vi "SI101_ACT_loop_n.vi"(0 "SI101_AverageReactorCoolantTemperature.lvclass in":refnum<class "SI101_AverageReactorCoolantTemperature.lvclass">, 1 "3 JEC10 CT001A XQ01":dbl, 2 "3 JEC20 CT001A XQ01":dbl, 3 "3 JEC30 CT001A XQ01":dbl, 4 "3 JEC40 CT001A XQ01":dbl, 5 "error in (no error)":errorcluster) -> (14 "SI101_AverageReactorCoolantTemperature.lvclass out":refnum<class "SI101_AverageReactorCoolantTemperature.lvclass">, 15 "JEC10CT001A":dbl, 16 "JEC20CT001A":dbl, 17 "JEC30CT001A":dbl, 18 "JEC40CT001A":dbl, 19 "error out":errorcluster)   [LabVIEW 2022 SP3, in "SI101_AverageReactorCoolantTemperature.lvclass"]
uses:
  SI101/SI101_AverageReactorCoolantTemperature.lvclass
  SI101/SI101_AverageReactorCoolantTemperature.lvclass/SI101_AverageReactorCoolantTemperature.ctl
panel:
  in  "Set Params":T1
  in  "Set Params 4":T1
  in  "Set Params 3":T1
  in  "Set Params 2":T1
  # "SI101"
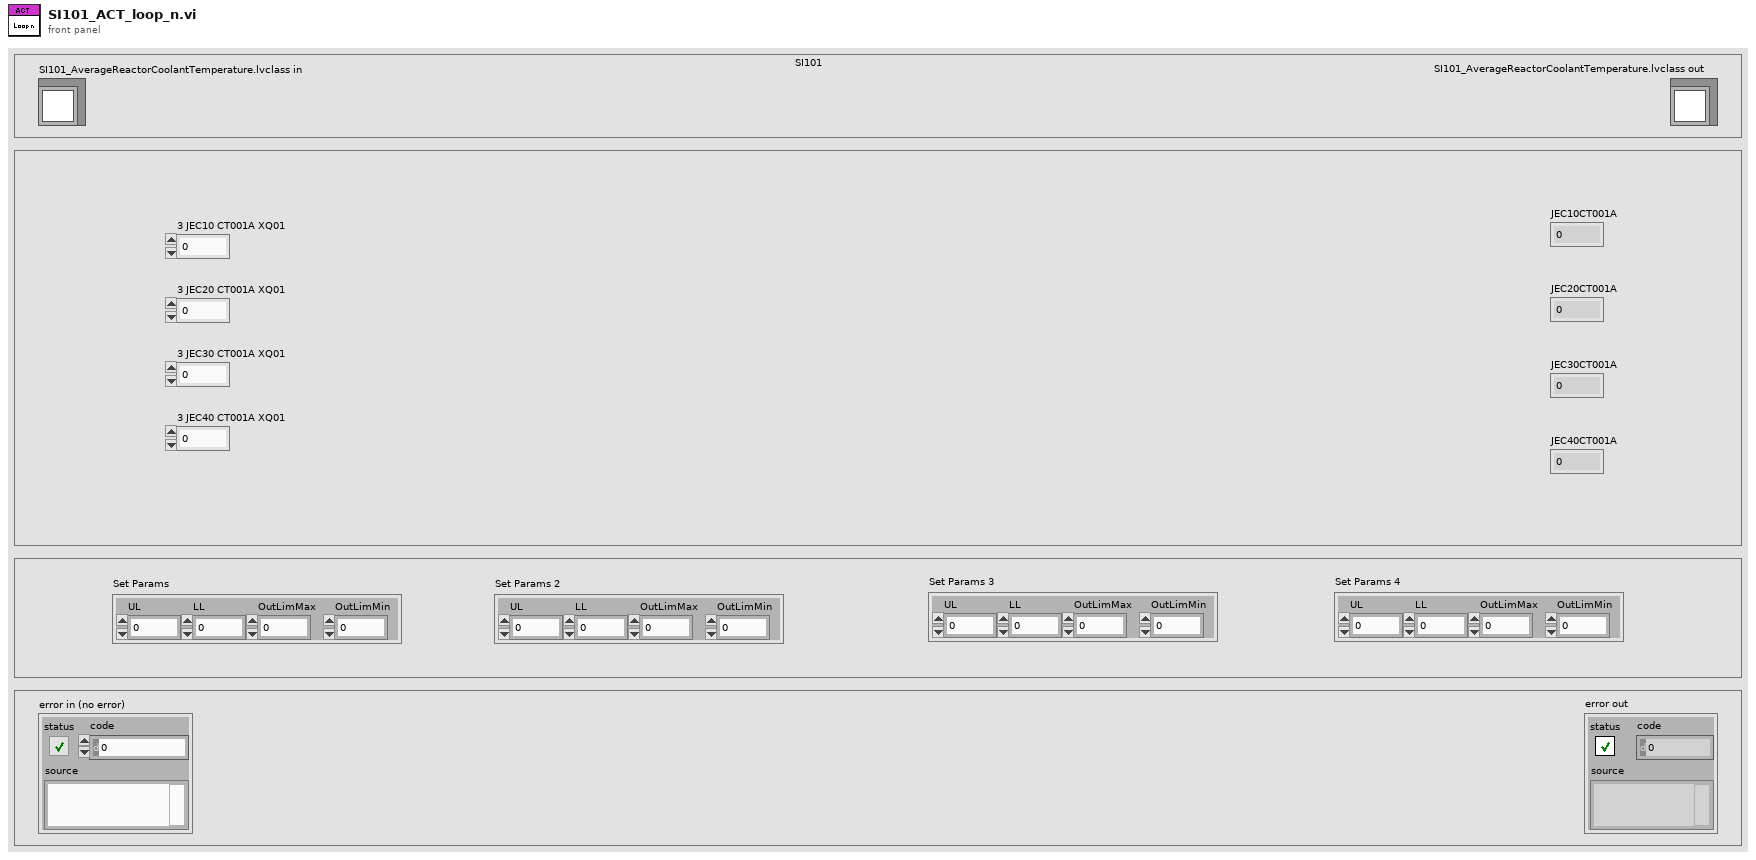
[diagram p1: front panel]
types:
  T1 = cluster{"UL":dbl, "LL":dbl, "OutLimMax":dbl, "OutLimMin":dbl}
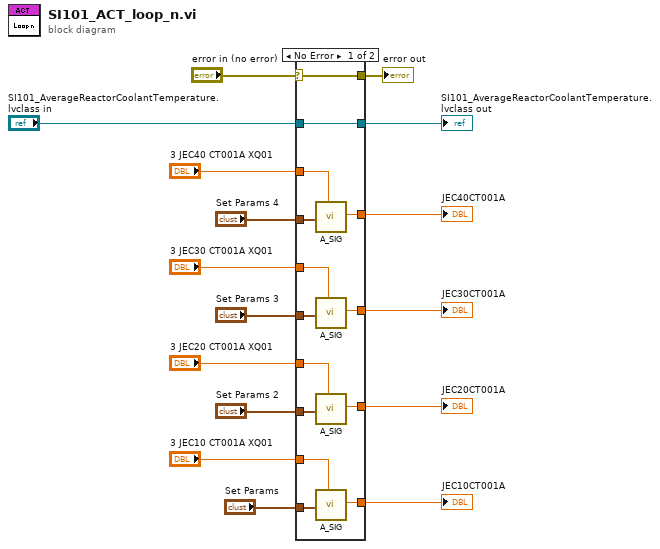
[diagram p0: block diagram]
diagram:
  n1 = case shown="No Error" "error in (no error)" {
    selector: "error in (no error)" -> [w30 w32]
    tunnel: [w30 w32] -> w15
    tunnel: "3 JEC20 CT001A XQ01" -> [w28 _]
    tunnel: "3 JEC10 CT001A XQ01" -> [w29 _]
    tunnel: "3 JEC30 CT001A XQ01" -> [w27 _]
    tunnel: "3 JEC40 CT001A XQ01" -> [w26 _]
    tunnel: "Set Params 2" -> [w25 _]
    tunnel: "Set Params 3" -> [w24 _]
    tunnel: "Set Params 4" -> [w23 _]
    tunnel: [w22 _] -> w7
    tunnel: [w21 _] -> w6
    tunnel: [w20 _] -> w5
    tunnel: [w19 _] -> w4
    tunnel: [w18 w31] -> w3
    tunnel: "SI101_AverageReactorCoolantTemperature.lvclass in" -> [w18 w31]
    tunnel: "Set Params" -> [w17 _]
    frame No Error {
      n2 = call "A_SIG.vi"("Set Params"=w23, "Input"=w26) -> ("A_SIG_out"=w19:dbl)  [unwired: 16 in, 1 out]
      n3 = call "A_SIG.vi"("Set Params"=w24, "Input"=w27) -> ("A_SIG_out"=w20:dbl)  [unwired: 16 in, 1 out]
      n4 = call "A_SIG.vi"("Set Params"=w25, "Input"=w28) -> ("A_SIG_out"=w21:dbl)  [unwired: 16 in, 1 out]
      n5 = call "A_SIG.vi"("Set Params"=w17, "Input"=w29) -> ("A_SIG_out"=w22:dbl)  [unwired: 16 in, 1 out]
    }
    frame Error {
    }
  }
  "error out" <- w15
  "SI101_AverageReactorCoolantTemperature.lvclass out" <- w3
  "JEC10CT001A" <- w7
  "JEC20CT001A" <- w6
  "JEC30CT001A" <- w5
  "JEC40CT001A" <- w4
